vi "Hardware Check.vi"() -> (1 "Data Acq Device":string, 2 "Data Directory Path":path, 3 "Has A/D board":bool)   [LabVIEW 2020]
doc: "Finds the NBMIO-16X board and the volume name.\nScott Hannahs, FBNML, Jan 1992"
uses:
  <vilib>/_DAQmxBase/Internals/DAQmxBase Register Map Strict Type Def.ctl
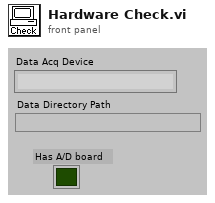
[diagram p1: front panel]
types:
  T1 = typedef "DAQmxBase Register Map Strict Type Def.ctl" = enum16{"none", "4452", "4472", "6110", "DIO32HS", "DIO96", "ESeries", "CFDAQ6004", "USB-92xx", "67xx", "SSeries", "MSeries", "USB-621x"}
  T2 = cluster{"Name":string, "Register Map":T1, "Index":u32}
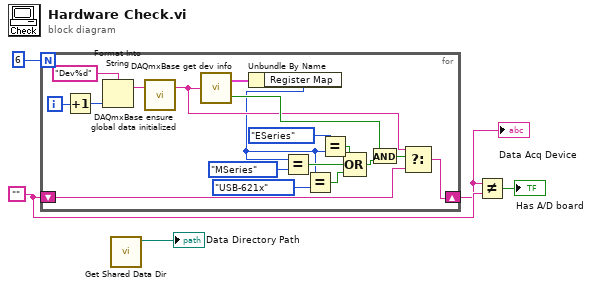
[diagram p0: block diagram]
diagram:
  w4 = ""
  n1 = for {
    N: 6 -> [_]
    shift-right: [w14] -> w3
    shift-left: w4 -> [w15]
    i -> [w23]
    n2 = Increment(x=w23) -> (x+1=w19:i32)
    n3 = Format Into String(format string="Dev%d", w19) -> (resulting string=w10:string)  [unwired: 2 in, 1 out]
    n4 = call <vilib>:"DAQmxBase ensure global data initialized.vi"("Task/Channel String in"=w10) -> ("Task/Channel String out"=w9:string)  [unwired: 1 in, 1 out]
    n5 = call <vilib>:"DAQmxBase get dev info.vi"("Device"=w9) -> ("Device Info"=w21:T2, "Exist?"=w17:bool)
    n6 = Unbundle By Name(w21) -> ("Register Map"=w7:T1)
    n7 = Equal?(x=w7, y=DAQmxBase_Register_Map_Strict_Type_Def."MSeries") -> (x = y?=w18:bool)
    n8 = Equal?(x=w7, y=DAQmxBase_Register_Map_Strict_Type_Def."USB-621x") -> (x = y?=w8:bool)
    n9 = Equal?(x=DAQmxBase_Register_Map_Strict_Type_Def."ESeries", y=w7) -> (x = y?=w12:bool)
    n10 = Compound Arithmetic op=OR(w12, w18, w8) -> (w13:bool)
    n11 = And(x=w17, y=w13) -> (x .and. y?=w16:bool)
    n12 = Select(t=w9, s=w16, f=w15) -> (s? t:f=w14:string)
  }
  "Data Acq Device" <- w3
  n13 = call "Get Shared Data Dir.vi"() -> ("Data Directory Path"=→"Data Directory Path":path)  [unwired: 2 in, 1 out]
  n14 = Not Equal?(x=w3, y=w4) -> (x != y?=→"Has A/D board":bool)
